vi "Rawdata_Imagedata_Analyzer.vi"() -> ()   [LabVIEW 2020]
uses:
  ctl/Image_Configuration.ctl
  ctl/Image_RAW_Bayer_Pattern.ctl
panel:
  out "Frame Size":i32
  out "Total Size":i64
  in  "stop":bool
  out "Image":T1(plugin-control)
  in  "Display":bool
  in  "Frame Index":i32
  in  "Bayer Pattern":T2=enum."BGGR (GBRG)"
  in  "Image Configuration":T3={"Width"=1920, "Height"=1536}
  out "error out":errorcluster
  out "Num of Meatadata":i64
  in  "Imagedata File Path":path
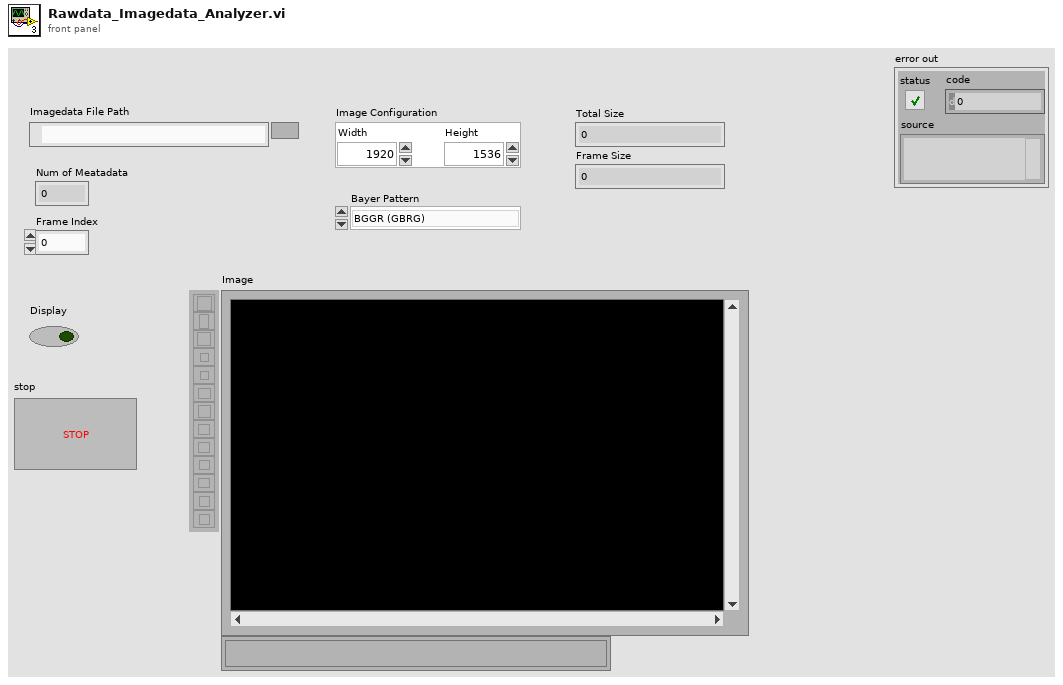
[diagram p1: front panel]
types:
  T1 = typedef "IMAQ Image.ctl" = refnum<image>
  T2 = typedef "Image_RAW_Bayer_Pattern.ctl" = enum16{"GBRG (BGGR)", "GRBG (RGGB)", "BGGR (GBRG)", "RGGB (GRBG)", "CRBC (RCCB)"}
  T3 = typedef "Image_Configuration.ctl" = cluster{"Width":i32, "Height":i32}
  T4 = enum16{"big-endian, network order", "native, host order", "little-endian"}
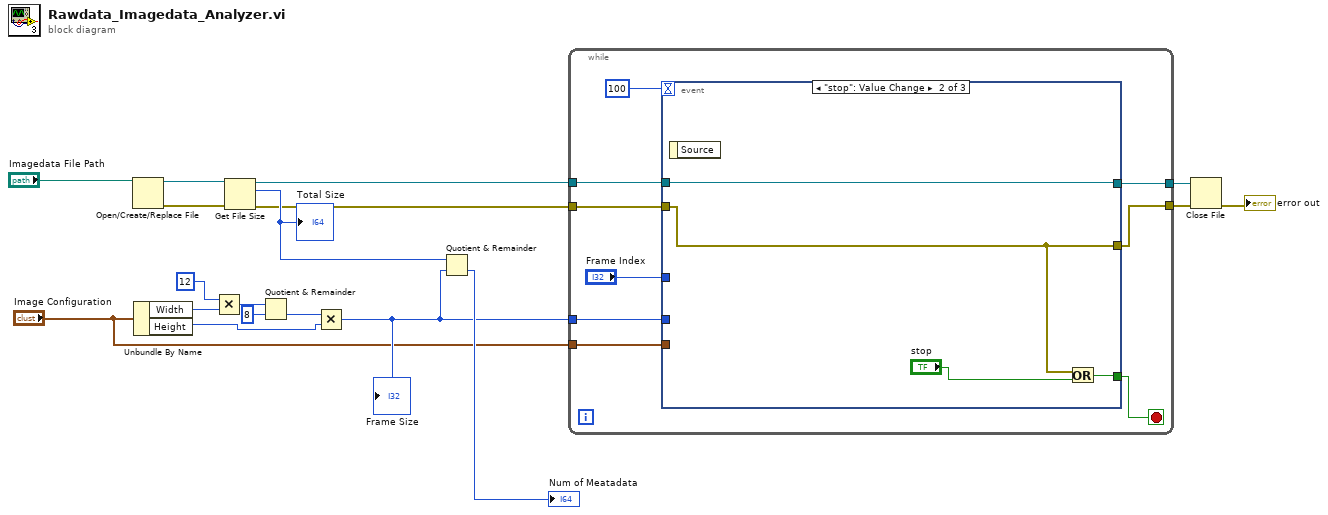
[diagram p0: block diagram]
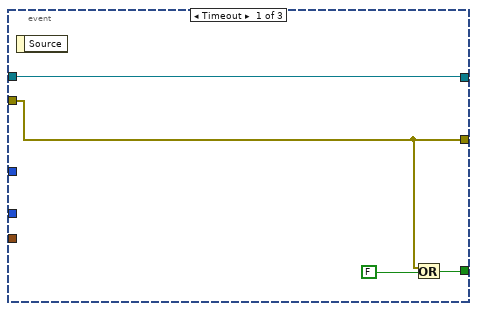
[diagram p2: hidden frame]
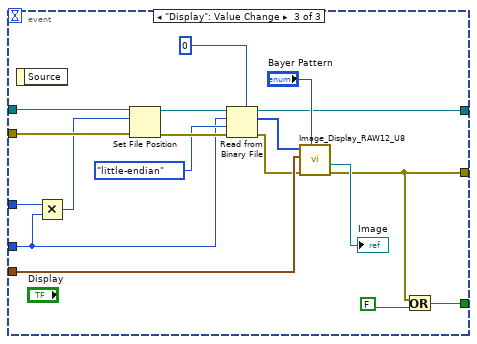
[diagram p3: hidden frame]
diagram:
  n1 = Open/Create/Replace File(file path (use dialog)="Imagedata File Path") -> (refnum out=w17:refnum<file>, error out=w16:errorcluster)  [unwired: 5 in, 1 out]
  n2 = Unbundle By Name("Image Configuration") -> ("Width"=w12:i32, "Height"=w7:i32)
  n3 = Multiply(x=12, y=w12) -> (x*y=w10:i32)
  n4 = Get File Size(file=w17, error in=w16) -> (refnum out=w4:refnum<file>, size (in bytes)=w15:i64, 0:w5:errorcluster)
  "Total Size" <- w15
  n5 = Quotient & Remainder(x=w10, y=8) -> (floor(x/y)=w8:i32)  [unwired: 1 out]
  n6 = Multiply(x=w8, y=w7) -> (x*y=w6:i32)
  "Frame Size" <- w6
  n7 = Quotient & Remainder(x=w15, y=w6) -> (floor(x/y)=→"Num of Meatadata":i64)  [unwired: 1 out]
  n8 = while {
    tunnel: w6 -> [w26]
    tunnel: w5 -> [w24]
    tunnel: w4 -> [w23]
    tunnel: "Image Configuration" -> [w22]
    tunnel: [w21] -> w2
    tunnel: [w20] -> w1
    stop <- w19 stop-if-true
    n9 = event shown="[1] \"stop\": Value Change" {
      selector: _ -> [_ _ _]
      dyn-events: _ -> [_ _ _]
      timeout: 100 -> [_ _ _]
      tunnel: w26 -> [_ _ w45]
      tunnel: "Frame Index" -> [_ _ w53]
      tunnel: w24 -> [w29 w33 w47]
      tunnel: w23 -> [w31 w35 w48]
      tunnel: w22 -> [_ _ w42]
      tunnel: [w29 w33 w37] -> w21
      tunnel: [w31 w35 w40] -> w20
      tunnel: [w30 w34 w36] -> w19
      event Timeout {
        n10 = event-data() -> ()  [unwired: 1 in, 1 out]
        n11 = Or(x=w29, y=FALSE) -> (x .or. y?=w30:bool)
      }
      event "stop": Value Change {
        n12 = event-data() -> ()  [unwired: 1 in, 1 out]
        n13 = Or(x=w33, y="stop") -> (x .or. y?=w34:bool)
      }
      event "Display": Value Change {
        n14 = event-data() -> ()  [unwired: 1 in, 1 out]
        n15 = Multiply(x=w53, y=w45) -> (x*y=w46:i32)
        n16 = Set File Position(offset (in bytes) (0)=w46, refnum=w48, error in=w47) -> (refnum out=w52:refnum<file>, error out=w51:errorcluster)  [unwired: 1 in]
        n17 = Read from Binary File(5:u8 0, 8:w51, 9:T4."little-endian" ("byte order (0:big-endian, network order)"), 10:w45, 11:w52) -> (0:w41:errorcluster, 2:w44:u8[], 3:w40:refnum<file>)  [unwired: 1 in, 1 out]
        n18 = call "Image_Display_RAW12_U8.vi"("Bayer Pattern"="Bayer Pattern", "error in (no error)"=w41, "Image Configuration"=w42, "RAW12 Frame (U8)"=w44) -> ("error out"=w37:errorcluster, "Image"=→"Image":T1)  [unwired: 4 in, 2 out]
        n19 = Or(x=w37, y=FALSE) -> (x .or. y?=w36:bool)
      }
    }
  }
  n20 = Close File(refnum=w1, error in=w2) -> (error out=→"error out":errorcluster)  [unwired: 1 out]
